vi "Model_v1.vi"(5 "state_variables":T1, 7 "model_v1_parameters":T2, 8 "init?":bool, 10 "assumed_U":bool, 11 "Control delay buffer":bool[](array[boolean])) -> (3 "Y_out":dbl)   [LabVIEW 2021, in "MBPOnOff_Controller.lvlib" / "Model_Predictor.lvclass"]
uses:
  Model_Predictor/Model_Predictor.lvclass
  Model_Predictor/typedefs/Model_v1_parameters.ctl
  Model_Predictor/typedefs/state_variables.ctl
panel:
  out "kLa_out":dbl
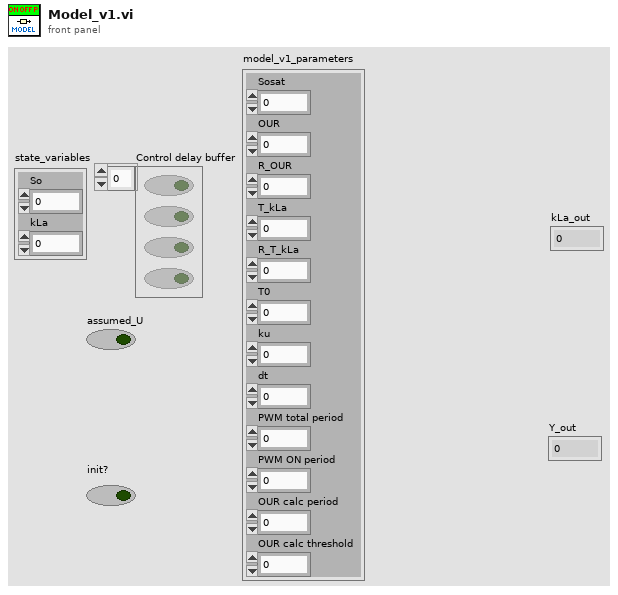
[diagram p1: front panel]
types:
  T1 = typedef "MBPOnOff_Controller.lvlib/Model_Predictor.lvclass/state_variables.ctl" = cluster{"So":dbl, "kLa":dbl}
  T2 = typedef "MBPOnOff_Controller.lvlib/Model_Predictor.lvclass/Model_v1_parameters.ctl" = cluster{"Sosat":dbl, "OUR":dbl, "R_OUR":dbl, "T_kLa":dbl, "R_T_kLa":dbl, "T0":dbl, "ku":dbl, "dt":dbl, "PWM total period":dbl, "PWM ON period":dbl, "OUR calc period":dbl, "OUR calc threshold":dbl}
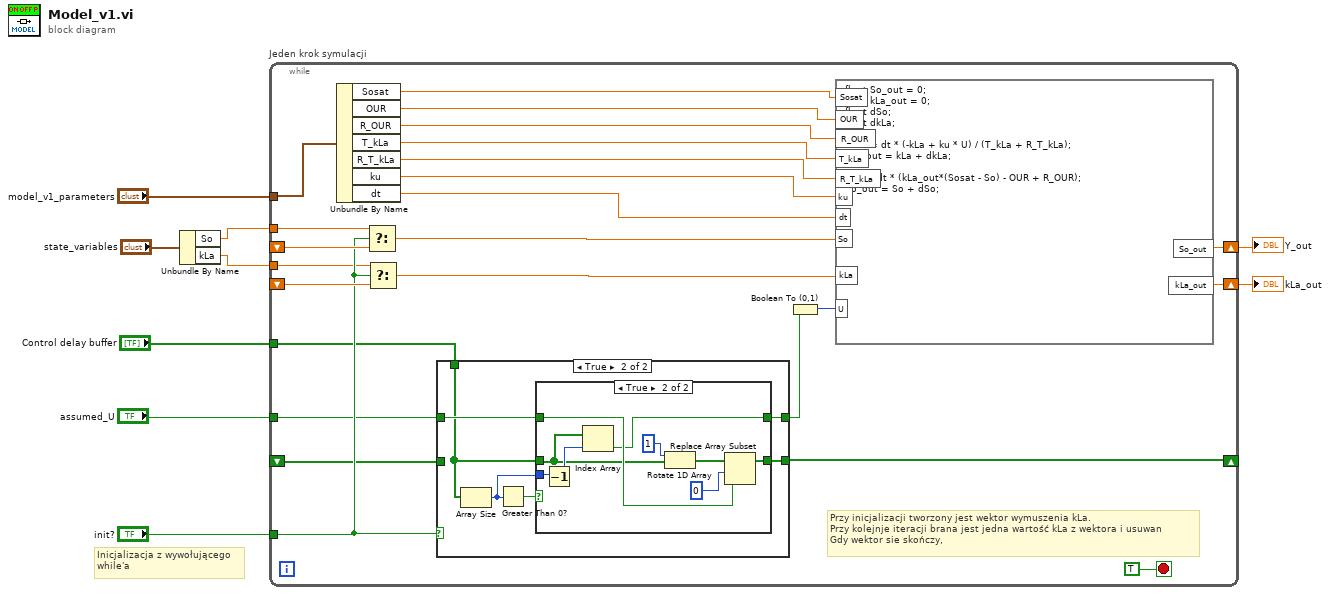
[diagram p0: block diagram]
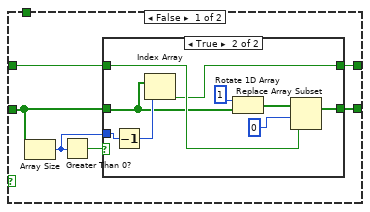
[diagram p2: hidden frame]
diagram:
  # "Inicjalizacja z wywołującego\nwhile'a"
  n1 = Unbundle By Name("state_variables") -> ("So"=w3:dbl, "kLa"=w2:dbl)
  n2 = while "Jeden krok symulacji" {
    shift-right: [w30] -> w9
    shift-left: _ -> [w27]
    tunnel: "model_v1_parameters" -> [w25]
    shift-right: [w29] -> w6
    shift-left: _ -> [w26]
    tunnel: "init?" -> [w24]
    tunnel: w3 -> [w32]
    tunnel: w2 -> [w23]
    shift-right: [w22] -> _
    shift-left: _ -> [w21]
    tunnel: "assumed_U" -> [w20]
    tunnel: "Control delay buffer" -> [w10]
    stop <- TRUE stop-if-true
    # "Przy inicjalizacji tworzony jest wektor wymuszenia kLa.\nPrzy kolejnje iteracji brana jest jedna wartość kLa z wektora i usuwan\nGdy wektor sie skończy,"
    n3 = Unbundle By Name(w25) -> ("Sosat"=w17:dbl, "OUR"=w16:dbl, "R_OUR"=w15:dbl, "T_kLa"=w14:dbl, "R_T_kLa"=w13:dbl, "ku"=w12:dbl, "dt"=w11:dbl)
    n4 = Select(t=w32, s=w24, f=w27) -> (s? t:f=w31:dbl)
    n5 = Select(t=w23, s=w24, f=w26) -> (s? t:f=w28:dbl)
    n6 = case shown="True" w24 {
      tunnel: [w39 w56] -> w22
      tunnel: w21 -> [w38 _]
      tunnel: w20 -> [w36 w54]
      tunnel: [w34 w55] -> w18
      tunnel: w10 -> [_ w52]
      frame False {
        n7 = Array Size(array=w38) -> (size(s)=w35:i32)
        n8 = Greater Than 0?(x=w35) -> (x > 0?=w37:bool)
        n9 = case shown="True" w37 {
          tunnel: [w41 w46] -> w39
          tunnel: w38 -> [w41 w42]
          tunnel: w36 -> [w40 w47]
          tunnel: w35 -> [_ w44]
          tunnel: [w40 w43] -> w34
          frame False {
          }
          frame True {
            n10 = Decrement(x=w44) -> (x-1=w45:i32)
            n11 = Index Array(array=w42, index=w45) -> (element=w43:bool)
            n12 = Rotate 1D Array(1:w42, 2:1 ("n")) -> (0:w49:bool[])
            n13 = Replace Array Subset(array=w49, new element=w47, index=0) -> (w46:bool[])
          }
        }
      }
      frame True {
        n14 = Array Size(array=w52) -> (size(s)=w51:i32)
        n15 = Greater Than 0?(x=w51) -> (x > 0?=w53:bool)
        n16 = case shown="True" w53 {
          tunnel: [w57 w67] -> w56
          tunnel: w54 -> [w58 w65]
          tunnel: [w58 w59] -> w55
          tunnel: w52 -> [w57 w61]
          tunnel: w51 -> [_ w64]
          frame False {
          }
          frame True {
            n17 = Decrement(x=w64) -> (x-1=w63:i32)
            n18 = Index Array(array=w61, index=w63) -> (element=w59:bool)
            n19 = Rotate 1D Array(1:w61, 2:1 ("n")) -> (0:w60:bool[])
            n20 = Replace Array Subset(array=w60, new element=w65, index=0) -> (w67:bool[])
          }
        }
      }
    }
    n21 = Boolean To (0,1)(Boolean=w18) -> (0, 1=w19:i16)
    n22 = formula code="float So_out = 0;\nfloat kLa_out = 0;\nfloat dSo;\nfloat dkLa;\n\ndkLa = dt * (-kLa + ku * U) / (T_kLa + R_T_kLa);\nkLa_out = kLa + dkLa;\n\ndSo = dt * (kLa_out*(Sosat - So) - OUR + R_OUR);\nSo_out = So + dSo;"("So"=w31, "kLa"=w28, "Sosat"=w17, "OUR"=w16, "T_kLa"=w14, "U"=w19, "R_OUR"=w15, "R_T_kLa"=w13, "ku"=w12, "dt"=w11) -> ("So_out"=w30:dbl, "kLa_out"=w29:dbl)
  }
  "Y_out" <- w9
  "kLa_out" <- w6
